vi "H5ObjInfoToLVH5ObjInfo.vi"(1 "H5O_info_t":T5 {"H5O_hdr_info_t"."mesg"."shared" format="%.0x"; "H5O_hdr_info_t"."mesg"."present" format="%.0x"; "H5O_hdr_info_t"."flags" format="%.0x"; "type" items=["H5O_TYPE_UNKNOWN"=-1, "H5O_TYPE_GROUP"=0, "H5O_TYPE_DATASET"=1, "H5O_TYPE_NAMED_DATATYPE"=2]}) -> (0 "LVH5O_info_t":T1 {"H5O_hdr_info_t"."mesg"."shared" format="%.0x"; "H5O_hdr_info_t"."mesg"."present" format="%.0x"; "H5O_hdr_info_t"."flags" format="%.0x"; "type" items=["H5O_TYPE_UNKNOWN"=-1, "H5O_TYPE_GROUP"=0, "H5O_TYPE_DATASET"=1, "H5O_TYPE_NAMED_DATATYPE"=2]})   [LabVIEW 2017]
uses:
  <vilib>/UPVI/lvhdf5/object.llb/H5O_info_t.ctl
  <vilib>/UPVI/lvhdf5/object.llb/H5O_type_t.ctl
  <vilib>/UPVI/lvhdf5/object.llb/H5O_hdr_info_t.ctl
  <vilib>/UPVI/lvhdf5/library.llb/H5_ih_info_t.ctl
  <vilib>/UPVI/lvhdf5/object.llb/LVH5O_info_t.ctl
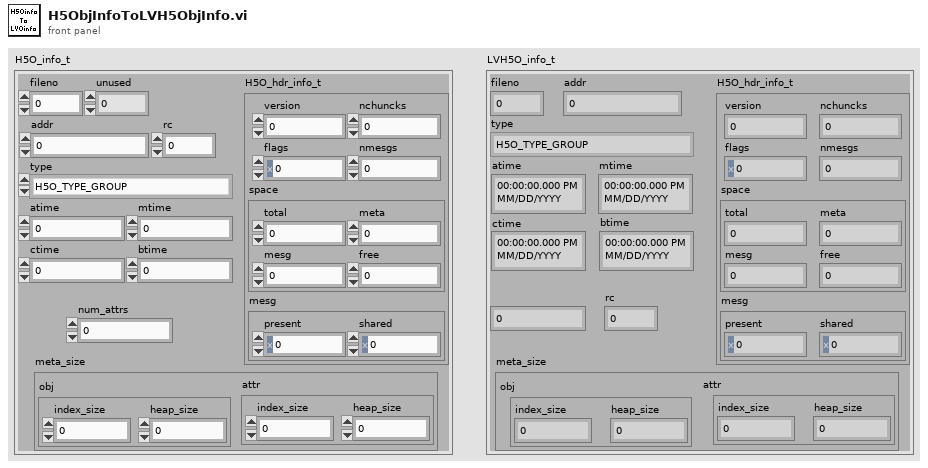
[diagram p1: front panel]
types:
  T1 = typedef "LVH5O_info_t.ctl" = cluster{"fileno":u32, "addr":u64, "type":T2, "rc":u32, "atime":timestamp, "mtime":timestamp, "ctime":timestamp, "btime":timestamp, "num_attrs":i64, "H5O_hdr_info_t":T3, "meta_size":cluster{"obj":T4, "attr":T4}}
  T2 = typedef "H5O_type_t.ctl" = i32
  T3 = typedef "H5O_hdr_info_t.ctl" = cluster{"version":u32, "nmesgs":u32, "nchuncks":u32, "flags":u32, "space":cluster{"total":u64, "meta":u64, "mesg":u64, "free":u64}, "mesg":cluster{"present":u64, "shared":u64}}
  T4 = typedef "H5_ih_info_t.ctl" = cluster{"index_size":u64, "heap_size":u64}
  T5 = typedef "H5O_info_t.ctl" = cluster{"fileno":u32, "unused":u32, "addr":u64, "type":T2, "rc":u32, "atime":i64, "mtime":i64, "ctime":i64, "btime":i64, "num_attrs":i64, "H5O_hdr_info_t":T3, "meta_size":cluster{"obj":T4, "attr":T4}}
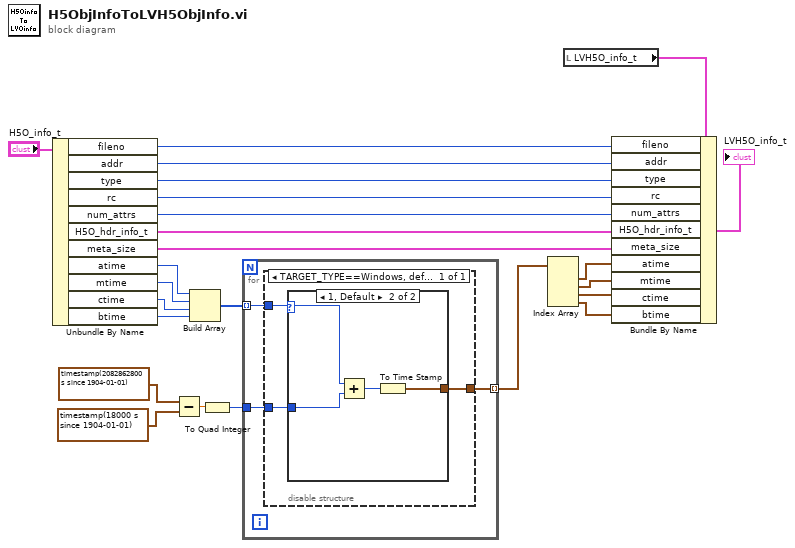
[diagram p0: block diagram]
diagram:
  n1 = Unbundle By Name("H5O_info_t") -> ("fileno"=w21:u32, "addr"=w20:u64, "type"=w19:T2, "rc"=w18:u32, "num_attrs"=w17:i64, "H5O_hdr_info_t"=w16:T3, "meta_size"=w15:cluster{"obj":T4, "attr":T4}, "atime"=w14:i64, "mtime"=w13:i64, "ctime"=w12:i64, "btime"=w11:i64)
  n2 = Subtract(x=timestamp(2082862800 s since 1904-01-01) ("time stamp"), y=timestamp(18000 s since 1904-01-01) ("time stamp")) -> (x-y=w7:dbl)
  n3 = Build Array(w14, w13, w12, w11) -> (w10:i64[])
  n4 = To Quad Integer(1:w7) -> (0:w6:i64)
  n5 = for {
    tunnel: w10 -> [w27] mode=indexing
    tunnel: w6 -> [w26]
    tunnel: [w25] -> w1 mode=indexing
    n6 = disable-structure shown="TARGET_TYPE==Windows, default" {
      disable-tunnel: w27 -> [w28]
      disable-tunnel: w26 -> [w30]
      disable-tunnel: [w29] -> w25
      frame condition #0 (active) {
        n7 = case shown="1, Default" w28 {
          selector: w28 -> [_ w31]
          tunnel: w30 -> [_ w34]
          tunnel: [_ w32] -> w29
          frame 0 {
          }
          frame 1, Default {
            n8 = Add(x=w31, y=w34) -> (x+y=w33:i64)
            n9 = To Time Stamp(1:w33) -> (0:w32:timestamp)
          }
        }
      }
    }
  }
  n10 = Index Array(array=w1) -> (element #1=w5:timestamp, element #2=w4:timestamp, element #3=w3:timestamp, element #4=w2:timestamp)  [unwired: 4 in]
  n11 = local read "LVH5O_info_t"() -> (w23:T1)
  n12 = Bundle By Name(cluster=w23, "fileno"=w21, "addr"=w20, "type"=w19, "rc"=w18, "num_attrs"=w17, "H5O_hdr_info_t"=w16, "meta_size"=w15, "atime"=w5, "mtime"=w4, "ctime"=w3, "btime"=w2) -> (→"LVH5O_info_t":T1)
